vi "RSZVB Set Source Combiner State.vi"(8 "error in (no error)":errorcluster {"code" format="%.0x"}, 9 "State (F: Off)":bool, 10 "Channel (1)":i32=1, 11 "VISA session":refnum<visa-resource-name>) -> (0 "error out":errorcluster {"code" format="%.0x"}, 3 "dup VISA session":refnum<visa-resource-name>)   [LabVIEW 2011]
doc: "This VI switches the source combiner for reference channel on or off.\n\n\nNotes:\n\n(1) This VI is available only with hardware option B11.\n\nRemote-control command(s):\nSOURce<Ch>:POWer:COMBiner ON | OFF"
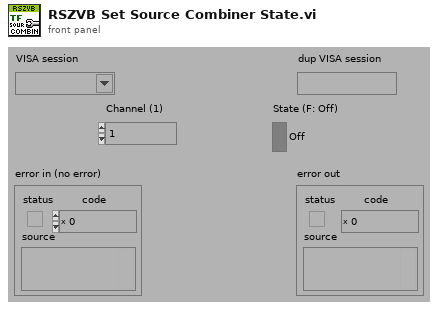
[diagram p1: front panel]
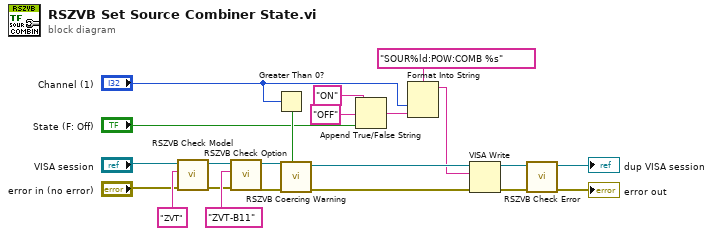
[diagram p0: block diagram]
diagram:
  n1 = call "RSZVB Check Model.vi"("error in (no error)"="error in (no error)", "Model"="ZVT" ("Options"), "VISA session"="VISA session") -> ("error out"=w4:errorcluster, "dup VISA session"=w2:refnum<visa-resource-name>)  [unwired: 7 in]
  n2 = call "RSZVB Check Option.vi"("error in (no error)"=w4, "Options"="ZVT-B11", "VISA session"=w2) -> ("error out"=w5:errorcluster, "dup VISA session"=w1:refnum<visa-resource-name>)  [unwired: 7 in]
  n3 = Greater Than 0?(x="Channel (1)") -> (x > 0?=w16:bool)
  n4 = call "RSZVB Coercing Warning.vi"("In Range?"=w16, "error in (no error)"=w5, "VISA session"=w1) -> ("error out"=w20:errorcluster, "dup VISA session"=w21:refnum<visa-resource-name>)  [unwired: 7 in]
  n5 = Append True/False String(1:"State (F: Off)", 2:"OFF", 3:"ON") -> (0:w13:string)  [unwired: 1 in]
  n6 = Format Into String(format string="SOUR%ld:POW:COMB %s", "Channel (1)", w13) -> (resulting string=w17:string)  [unwired: 2 in, 1 out]
  n7 = VISA Write(VISA resource name=w21, write buffer=w17, error in (no error)=w20) -> (VISA resource name out=w18:refnum<visa-resource-name>, error out=w19:errorcluster)  [unwired: 1 out]
  n8 = call "RSZVB Check Error.vi"("error in (no error)"=w19, "VISA session"=w18) -> ("error out"=→"error out":errorcluster, "dup VISA session"=→"dup VISA session":refnum<visa-resource-name>)  [unwired: 8 in]
